vi "LoadAdjust_WithPosition.vi"(7 "Current Position":dbl=2.0 min=0.0 max=2.0 step=0.01, 9 "y":i16, 10 "Load Curve":dbl[][](array[numeric]), 11 "Queue in":refnum<queue>) -> (1 "sum":i16)   [LabVIEW 2026, in "Acquisition.lvlib"]
uses:
  Acquisition.lvlib
  support/Message Queue/Message Cluster.ctl
  support/Message Queue/Enqueue Message (Single).vi
  support/Message Queue/Message Queue.lvlib
panel:
  out "Boolean 2":bool
  out "Brake Torque":dbl
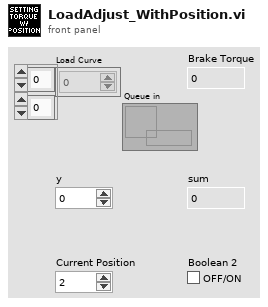
[diagram p1: front panel]
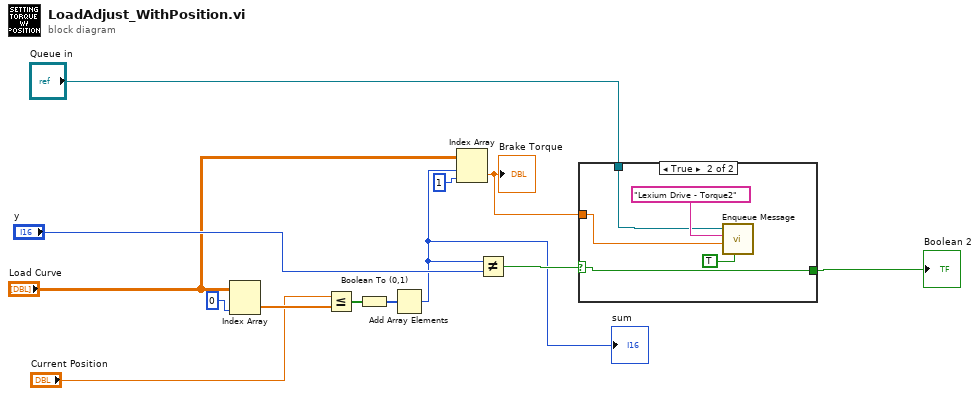
[diagram p0: block diagram]
diagram:
  n1 = Index Array(array="Load Curve", index (col)=0 ("index (row)")) -> (element=w5:dbl[])  [unwired: 1 in]
  n2 = Less Or Equal?(x="Current Position", y=w5) -> (x <= y?=w8:bool[])
  n3 = Boolean To (0,1)(Boolean=w8) -> (0, 1=w9:i16[])
  n4 = Add Array Elements(numeric array=w9) -> (sum=w10:i16)
  "sum" <- w10
  n5 = Index Array(array="Load Curve", index (row)=w10, index (col)=1 ("disabled index (col)")) -> (element=w2:dbl)
  "Brake Torque" <- w2
  n6 = Not Equal?(x=w10, y="y") -> (x != y?=w11:bool)
  n7 = case shown="True" w11 {
    selector: w11 -> [w14 w19]
    tunnel: [w14 w19] -> w12
    tunnel: w2 -> [_ w16]
    tunnel: "Queue in" -> [_ w15]
    frame False {
    }
    frame True {
      n8 = call-poly "Enqueue Message.vi"("Priority Message? (F)"=TRUE, "Message Data"=w16, "Message"="Lexium Drive - Torque2", "Message Queue"=w15) -> ()  [unwired: 6 in, 2 out]
    }
  }
  "Boolean 2" <- w12
